vi "DT_Ain_States.vi"() -> ()   [LabVIEW 2011]
uses:
  <userlib>/LV-Link3/PolySubVIs/DtCreateAinChan.vi
  <userlib>/LV-Link3/PolySubVIs/DtOLTimingSetInput.vi
  <userlib>/LV-Link3/PolySubVIs/DtOLReadMultiple2D.vi
panel:
  out "Actual Number of Channels":u32
  out "Num Samples Per Channel Read":i32
  out "Num Channels Read":i32
  in  "Tab Control":T1(tab)
  in  "Select":u32
  out "Number of Devices":u32
  out "Device Name":string
  in  "Select Device":bool
  in  "Sample Mode":enum16{"Finite Samples", "Continuous Samples"}(ring)
  in  "Sample Freq (Hz)":dbl=1000.0
  in  "Channel Type":i32(ring)=100 items=["SingleEnded"=100, "Differential"=101]
  in  "Channel Selection":string="Ain 0"
  in  "Timing":T2(ring)
  in  "Num Buffers":u32=8
  out "Actual Sample Freq":dbl
  out "Buffer Size":u32
  in  "Configure":bool
  out "Waveform Graph":dbl[][](graph)
  in  "Start Aquisition":bool
  in  "Stop Acquisition":bool
  in  "Exit Application":bool
  in  "error in (no error)":errorcluster
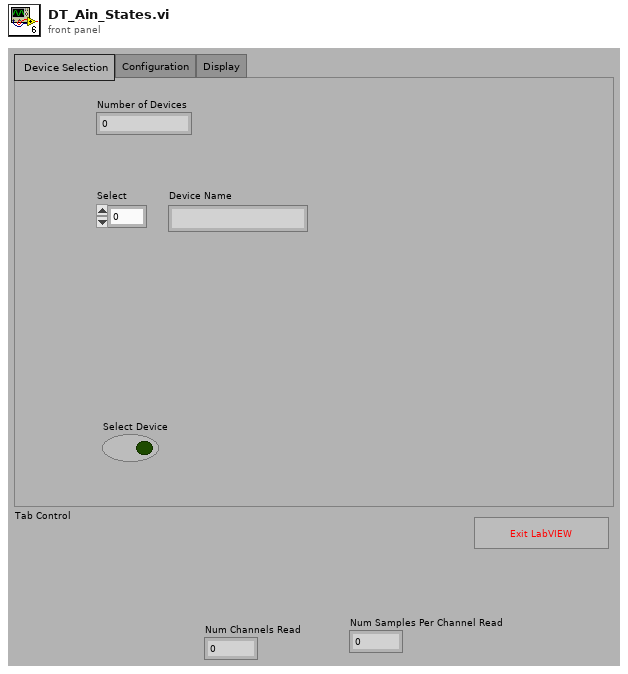
[diagram p1: front panel]
types:
  T1 = enum32{" Device Selection", "Configuration", "Display"}
  T2 = enum32{"Internal Clock", "External Clock", "No Timing"}
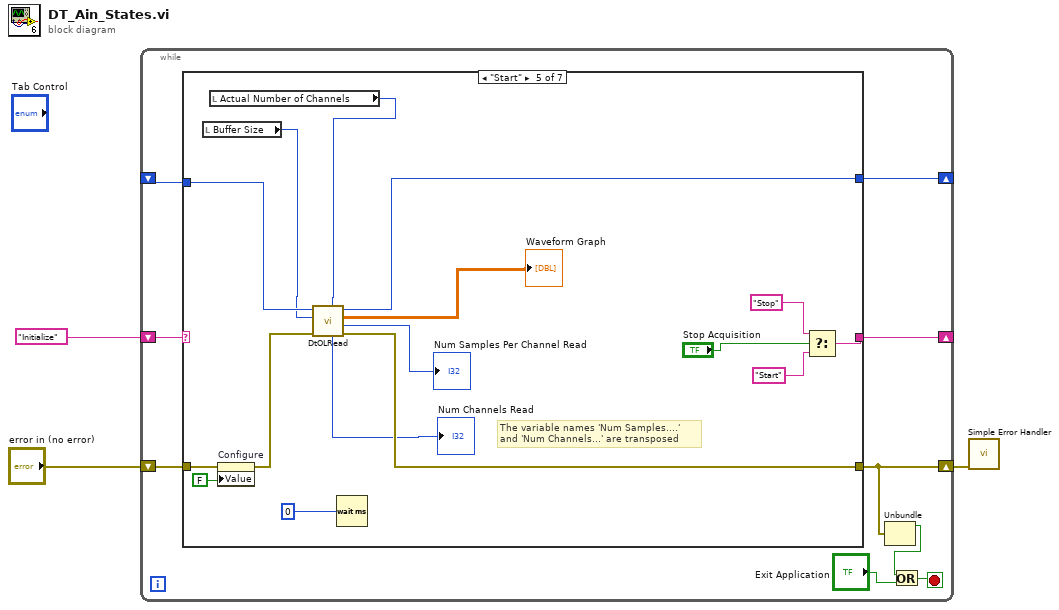
[diagram p0: block diagram]
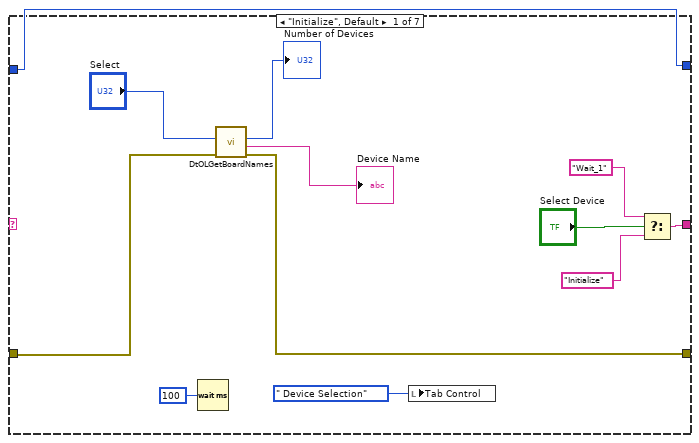
[diagram p2: hidden frame]
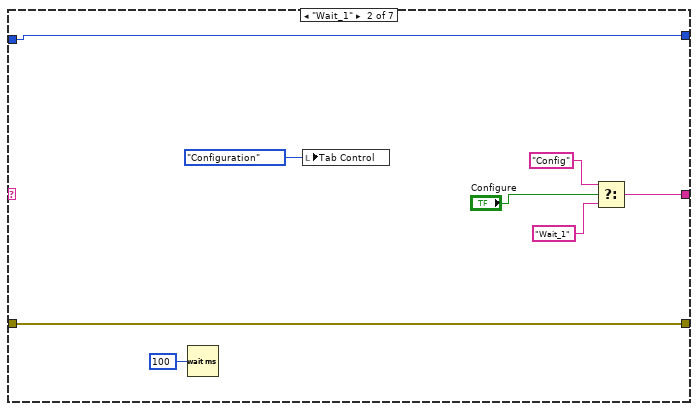
[diagram p3: hidden frame]
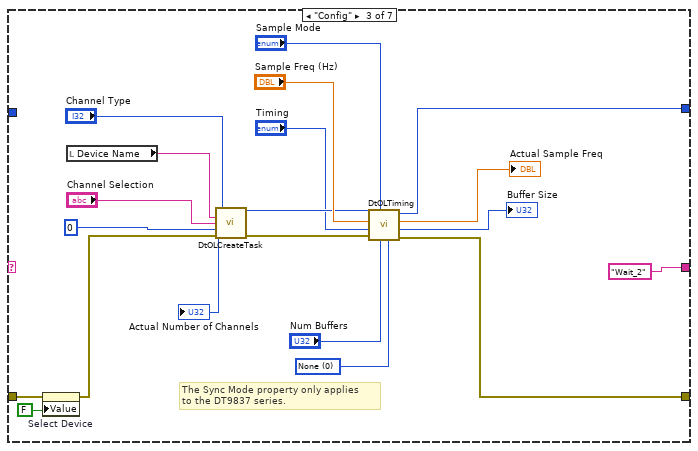
[diagram p4: hidden frame]
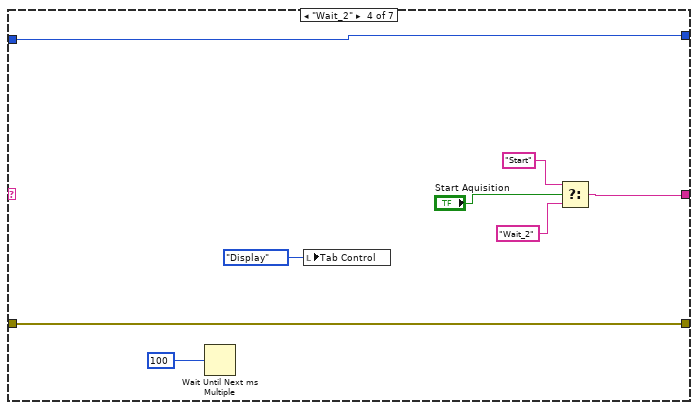
[diagram p5: hidden frame]
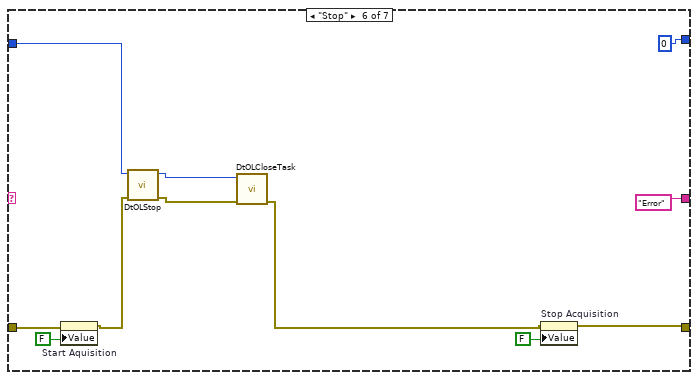
[diagram p6: hidden frame]
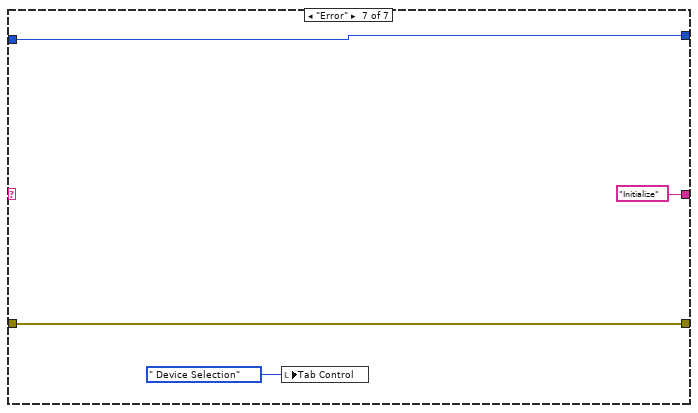
[diagram p7: hidden frame]
diagram:
  n1 = while {
    shift-right: [w7] -> w1
    shift-left: "error in (no error)" -> [w12]
    shift-right: [w10] -> _
    shift-left: "Initialize" ("String") -> [w11]
    shift-right: [w9] -> _
    shift-left: _ -> [w8]
    stop <- w6 stop-if-true
    n2 = case shown="\"Start\"" w11 {
      tunnel: w12 -> [w24 w28 w33 w59 w64 w80 w90]
      tunnel: [w17 w29 "Wait_2" ("f") w54 w71 "Error" ("String") "Initialize" ("String")] -> w10
      tunnel: [w21 w28 w39 w59 w74 w77 w90] -> w7
      tunnel: [w15 w27 w43 w58 w73 0 ("Task out") w89] -> w9
      tunnel: w8 -> [w15 w27 _ w58 w75 w86 w89]
      frame "Initialize", Default {
        n3 = Wait (ms)(milliseconds to wait=u32 100) -> ()  [unwired: 1 out]
        n4 = call <userlib>:"DtOLGetBoardNames.vi"("error in (no error)"=w24, "Select Board"="Select") -> ("error out"=w21:errorcluster, "Board Name"=→"Device Name":string, "Number of boards"=→"Number of Devices":u32)  [unwired: 7 in]
        n5 = local write "Tab Control"(T1." Device Selection" ("Tab Control")) -> ()
        n6 = Select(t="Wait_1" ("String"), s="Select Device", f="Initialize" ("String")) -> (s? t:f=w17:string)
      }
      frame "Wait_1" {
        n7 = Wait (ms)(milliseconds to wait=u32 100) -> ()  [unwired: 1 out]
        n8 = local write "Tab Control"(T1."Configuration" ("Tab Control")) -> ()
        n9 = Select(t="Config" ("String"), s="Configure", f="Wait_1") -> (s? t:f=w29:string)
      }
      frame "Config" {
        w41 = 0 items=["None", "Master", "Slave"] ("Sync Mode[DT9837 series only]")
        # "The Sync Mode property only applies\nto the DT9837 series."
        n10 = property on="Select Device" class="Bool (strict)"(error in=w33, "Value"=FALSE ("Select Device")) -> (error out=w34:errorcluster)  [unwired: 1 in, 1 out]
        n11 = local read "Device Name"() -> (w52:string)
        n12 = call-poly <userlib>:"DtOLCreateTask.vi"("Channel Type"="Channel Type", "Board Name"=w52, "Channel"="Channel Selection", "Element"=u32 0, "error in (no error)"=w34) -> ("Task out"=w47:i32, "Actual Number of Channels"=→"Actual Number of Channels":u32, "error out"=w49:errorcluster)  [unwired: 8 in]
        n13 = call-poly <userlib>:"DtOLTiming.vi"("Sync Mode"=w41, "Num Buffers"="Num Buffers", "Sample Mode"="Sample Mode", "error in (no error)"=w49, "Timing"="Timing", "Sample Freq (Hz)"="Sample Freq (Hz)", "Task in"=w47) -> ("error out"=w39:errorcluster, "Buffer Size"=→"Buffer Size":u32, "Actual Sample Freq"=→"Actual Sample Freq":dbl, "Task out"=w43:i32)  [unwired: 1 in]
      }
      frame "Wait_2" {
        n14 = Wait Until Next ms Multiple(millisecond multiple=u32 100) -> ()  [unwired: 1 out]
        n15 = local write "Tab Control"(T1."Display" ("Tab Control")) -> ()
        n16 = Select(t="Start" ("String"), s="Start Aquisition", f="Wait_2") -> (s? t:f=w54:string)
      }
      frame "Start" {
        # "The variable names 'Num Samples....' \nand 'Num Channels...' are transposed"
        n17 = local read "Buffer Size"() -> (w61:u32)
        n18 = local read "Actual Number of Channels"() -> (w62:u32)
        n19 = property on="Configure" class="Bool (strict)"(error in=w64, "Value"=FALSE ("Configure")) -> (error out=w65:errorcluster)  [unwired: 1 in, 1 out]
        n20 = call-poly <userlib>:"DtOLRead.vi"("Number Chan to Read"=w62, "error in (no error)"=w65, "Samples Per Channel"=w61, "Task in"=w75) -> ("error out"=w74:errorcluster, "Num Samples Per Channel Read"=→"Num Samples Per Channel Read":i32, "2D Data out"=→"Waveform Graph":dbl[][], "Task out"=w73:i32, "Num Channels Read"=→"Num Channels Read":i32)  [unwired: 3 in]
        n21 = Wait (ms)(milliseconds to wait=u32 0) -> ()  [unwired: 1 out]
        n22 = Select(t="Stop" ("String"), s="Stop Acquisition", f="Start") -> (s? t:f=w71:string)
      }
      frame "Stop" {
        n23 = property on="Start Aquisition" class="Bool (strict)"(error in=w80, "Value"=FALSE ("Start Aquisition")) -> (error out=w81:errorcluster)  [unwired: 1 in, 1 out]
        n24 = call <userlib>:"DtOLStop.vi"("error in (no error)"=w81, "Task in"=w86) -> ("error out"=w84:errorcluster, "Task out"=w85:i32)  [unwired: 8 in]
        n25 = call <userlib>:"DtOLCloseTask.vi"("Error in"=w84, "Task in"=w85) -> ("Error Out"=w78:errorcluster)  [unwired: 9 in]
        n26 = property on="Stop Acquisition" class="Bool (strict)"(error in=w78, "Value"=FALSE ("Stop Acquisition")) -> (error out=w77:errorcluster)  [unwired: 1 in, 1 out]
      }
      frame "Error" {
        n27 = local write "Tab Control"(T1." Device Selection" ("Tab Control")) -> ()
      }
    }
    n28 = Unbundle(w7) -> ("status"=w5:bool)  [unwired: 2 out]
    n29 = Or(x=w5, y="Exit Application") -> (x .or. y?=w6:bool)
  }
  n30 = call <vilib>:"Simple Error Handler.vi"("error in (no error)"=w1) -> ()  [unwired: 4 in, 5 out]
